vi "blinking lights 2.vi"() -> ()   [LabVIEW 2015]
panel:
  in  "stop":bool
  out "Boolean 1":bool
  out "Boolean 5":bool
  out "Boolean 4":bool
  out "Boolean 3":bool
  out "Boolean 2":bool
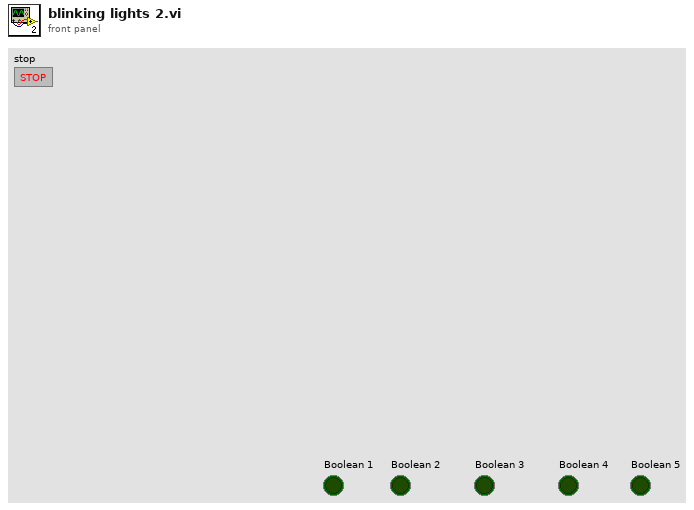
[diagram p1: front panel]
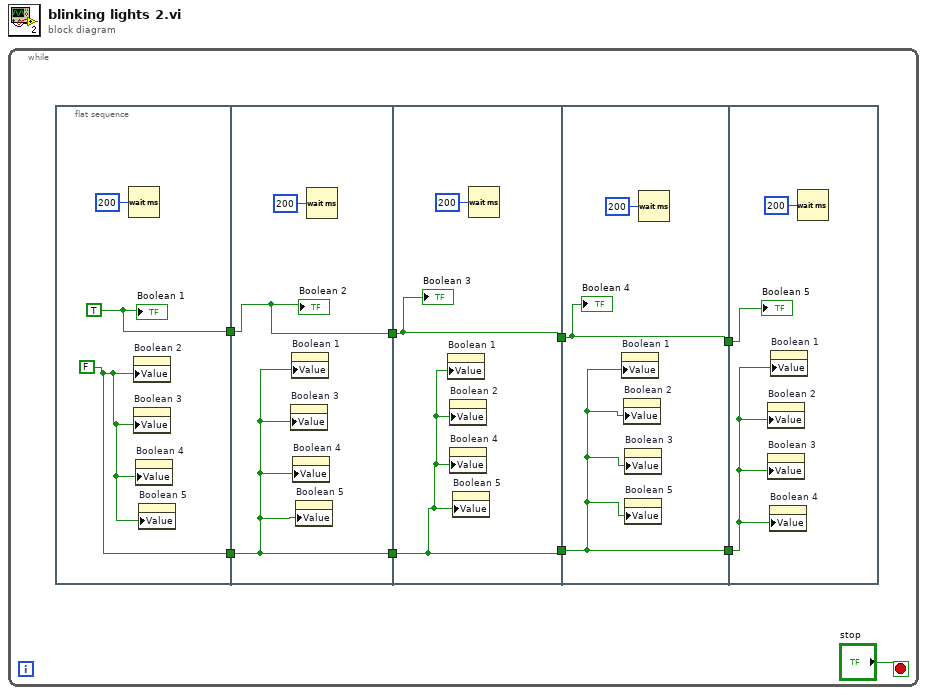
[diagram p0: block diagram]
diagram:
  n1 = while {
    stop <- "stop" stop-if-true
    n2 = flat-sequence {
      tunnel: [w11] -> w9
      tunnel: [w10] -> w4
      tunnel: w9 -> [w14]
      tunnel: [w14] -> w8
      tunnel: w4 -> [w13]
      tunnel: [w13] -> w3
      tunnel: w8 -> [w17]
      tunnel: [w17] -> w7
      tunnel: w3 -> [w16]
      tunnel: [w16] -> w2
      tunnel: w7 -> [w20]
      tunnel: [w20] -> w6
      tunnel: w2 -> [w19]
      tunnel: [w19] -> w1
      tunnel: w6 -> [w23]
      tunnel: w1 -> [w22]
      frame #0 {
        w10 = FALSE
        w11 = TRUE
        n3 = Wait (ms)(milliseconds to wait=u32 200) -> ()  [unwired: 1 out]
        n4 = property on="Boolean 2" class="Bool (strict)"("Value"=w10) -> ()  [unwired: 2 in, 2 out]
        n5 = property on="Boolean 3" class="Bool (strict)"("Value"=w10) -> ()  [unwired: 2 in, 2 out]
        n6 = property on="Boolean 4" class="Bool (strict)"("Value"=w10) -> ()  [unwired: 2 in, 2 out]
        n7 = property on="Boolean 5" class="Bool (strict)"("Value"=w10) -> ()  [unwired: 2 in, 2 out]
        "Boolean 1" <- w11
      }
      frame #1 {
        n8 = property on="Boolean 3" class="Bool (strict)"("Value"=w13) -> ()  [unwired: 2 in, 2 out]
        n9 = property on="Boolean 1" class="Bool (strict)"("Value"=w13) -> ()  [unwired: 2 in, 2 out]
        n10 = property on="Boolean 4" class="Bool (strict)"("Value"=w13) -> ()  [unwired: 2 in, 2 out]
        n11 = property on="Boolean 5" class="Bool (strict)"("Value"=w13) -> ()  [unwired: 2 in, 2 out]
        n12 = Wait (ms)(milliseconds to wait=u32 200) -> ()  [unwired: 1 out]
        "Boolean 2" <- w14
      }
      frame #2 {
        n13 = property on="Boolean 1" class="Bool (strict)"("Value"=w16) -> ()  [unwired: 2 in, 2 out]
        n14 = property on="Boolean 2" class="Bool (strict)"("Value"=w16) -> ()  [unwired: 2 in, 2 out]
        n15 = property on="Boolean 4" class="Bool (strict)"("Value"=w16) -> ()  [unwired: 2 in, 2 out]
        n16 = property on="Boolean 5" class="Bool (strict)"("Value"=w16) -> ()  [unwired: 2 in, 2 out]
        n17 = Wait (ms)(milliseconds to wait=u32 200) -> ()  [unwired: 1 out]
        "Boolean 3" <- w17
      }
      frame #3 {
        n18 = property on="Boolean 1" class="Bool (strict)"("Value"=w19) -> ()  [unwired: 2 in, 2 out]
        n19 = property on="Boolean 2" class="Bool (strict)"("Value"=w19) -> ()  [unwired: 2 in, 2 out]
        n20 = property on="Boolean 3" class="Bool (strict)"("Value"=w19) -> ()  [unwired: 2 in, 2 out]
        n21 = property on="Boolean 5" class="Bool (strict)"("Value"=w19) -> ()  [unwired: 2 in, 2 out]
        n22 = Wait (ms)(milliseconds to wait=u32 200) -> ()  [unwired: 1 out]
        "Boolean 4" <- w20
      }
      frame #4 {
        n23 = property on="Boolean 2" class="Bool (strict)"("Value"=w22) -> ()  [unwired: 2 in, 2 out]
        n24 = property on="Boolean 3" class="Bool (strict)"("Value"=w22) -> ()  [unwired: 2 in, 2 out]
        n25 = property on="Boolean 4" class="Bool (strict)"("Value"=w22) -> ()  [unwired: 2 in, 2 out]
        n26 = property on="Boolean 1" class="Bool (strict)"("Value"=w22) -> ()  [unwired: 2 in, 2 out]
        n27 = Wait (ms)(milliseconds to wait=u32 200) -> ()  [unwired: 1 out]
        "Boolean 5" <- w23
      }
    }
  }
